vi "sample obtain bucket get object.vi"() -> ()   [LabVIEW 2015]
uses:
  GET Object Result Parameters.ctl
  Core/HTTP Request/AWS Credentials.ctl
  GET Object Request Parameters.ctl
  Core/Request Range.ctl
  Bucket/Bucket.lvclass
  Core/HTTP Request/HTTP Request.lvclass
  Core/NI_AWS_Core.lvlib
  NI_AWS_S3.lvlib
panel:
  out "GetObjectResult":T1
  out "Object Data":string
  out "error out":errorcluster
  in  "Bucket name":string="bpreis-test-96"
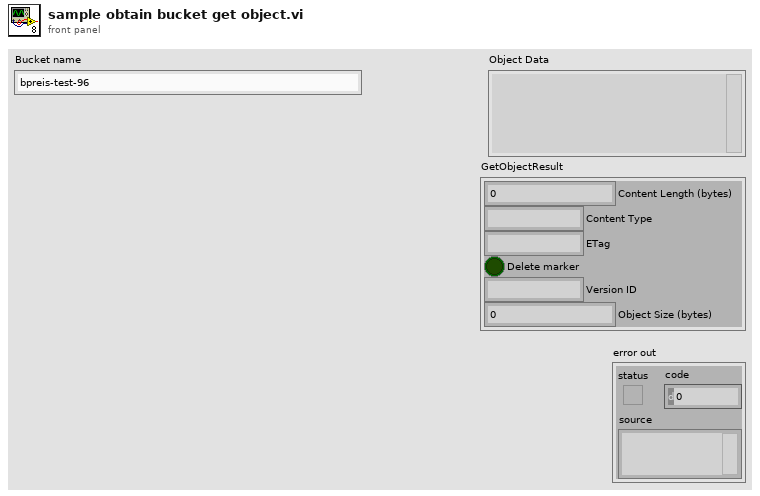
[diagram p1: front panel]
types:
  T1 = typedef "NI_AWS_S3.lvlib/GET Object Result Parameters.ctl" = cluster{"Content Length (bytes)":u64, "Content Type":string, "ETag":string, "Delete marker":bool, "Version ID":string, "Object Size (bytes)":u64}
  T2 = typedef "NI_AWS_S3.lvlib/GET Object Request Parameters.ctl" = cluster{"Range":T3, "If Modified Since":timestamp, "If Unmodified Since":timestamp, "Matching ETag":string, "Nonmatching ETag":string}
  T3 = typedef "NI_AWS_Core.lvlib/Request Range.ctl" = cluster{"Start":i64, "Length":i64}
  T4 = typedef "NI_AWS_Core.lvlib/HTTP Request.lvclass/AWS Credentials.ctl" = cluster{"Access Key":string, "Secret Key":string}
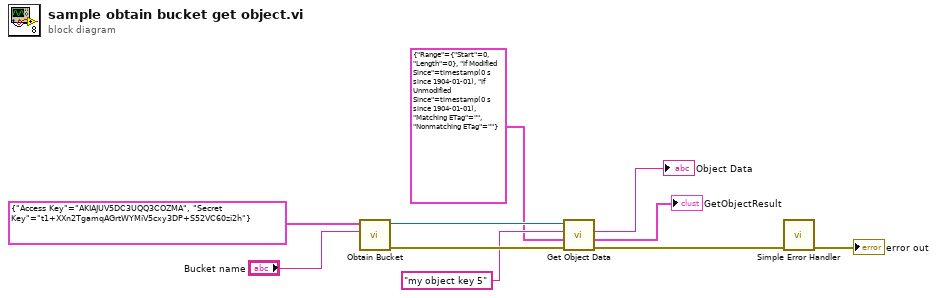
[diagram p0: block diagram]
diagram:
  n1 = call "Obtain Bucket.vi"("Bucket name"="Bucket name", "AWS Credentials"=T4 {"Access Key"="AKIAJUV5DC3UQQ3COZMA", "Secret Key"="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"}) -> ("error out"=w10:errorcluster, "Bucket"=w6:refnum<class "Bucket.lvclass">)  [unwired: 8 in]
  n2 = call "Get Object Data.vi"("error in (no error)"=w10, "Request Parameters"=T2 {"Range"={"Start"=0, "Length"=0}, "If Modified Since"=timestamp(0 s since 1904-01-01), "If Unmodified Since"=timestamp(0 s since 1904-01-01), "Matching ETag"="", "Nonmatching ETag"=""}, "Object Key"="my object key 5", "Bucket in"=w6) -> ("error out"=w5:errorcluster, "GetObjectResult"=→"GetObjectResult":T1, "Object Data"=→"Object Data":string)  [unwired: 4 in, 1 out]
  n3 = call <vilib>:"Simple Error Handler.vi"("error in (no error)"=w5) -> ("error out"=→"error out":errorcluster)  [unwired: 4 in, 4 out]
